vi "Get Ctrl Ref to Connect Unflatten Node.vi"(0 "VI Ref In":refnum<vi>, 5 "JSON String":string, 11 "Error In":errorcluster) -> (4 "Control Terminal References":T1[](array[typedef]), 15 "Error Out":errorcluster)   [LabVIEW 2019, in "JsonToCluster.lvlib"]
doc: "This VI gets control references to connect with unflatten from json string node"
uses:
  JsonToCluster.lvlib
  _Controls/Control Terminal Reference.ctl
  <vilib>/Utility/miscctls.llb/LVPositionTypeDef.ctl
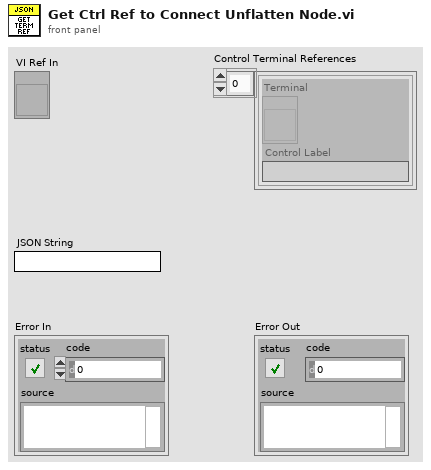
[diagram p1: front panel]
types:
  T1 = typedef "JsonToCluster.lvlib/Control Terminal Reference.ctl" = cluster{"Terminal":refnum<vi>, "Control Label":string}
  T2 = typedef "LVPositionTypeDef.ctl" = cluster{"Left":i32, "Top":i32}
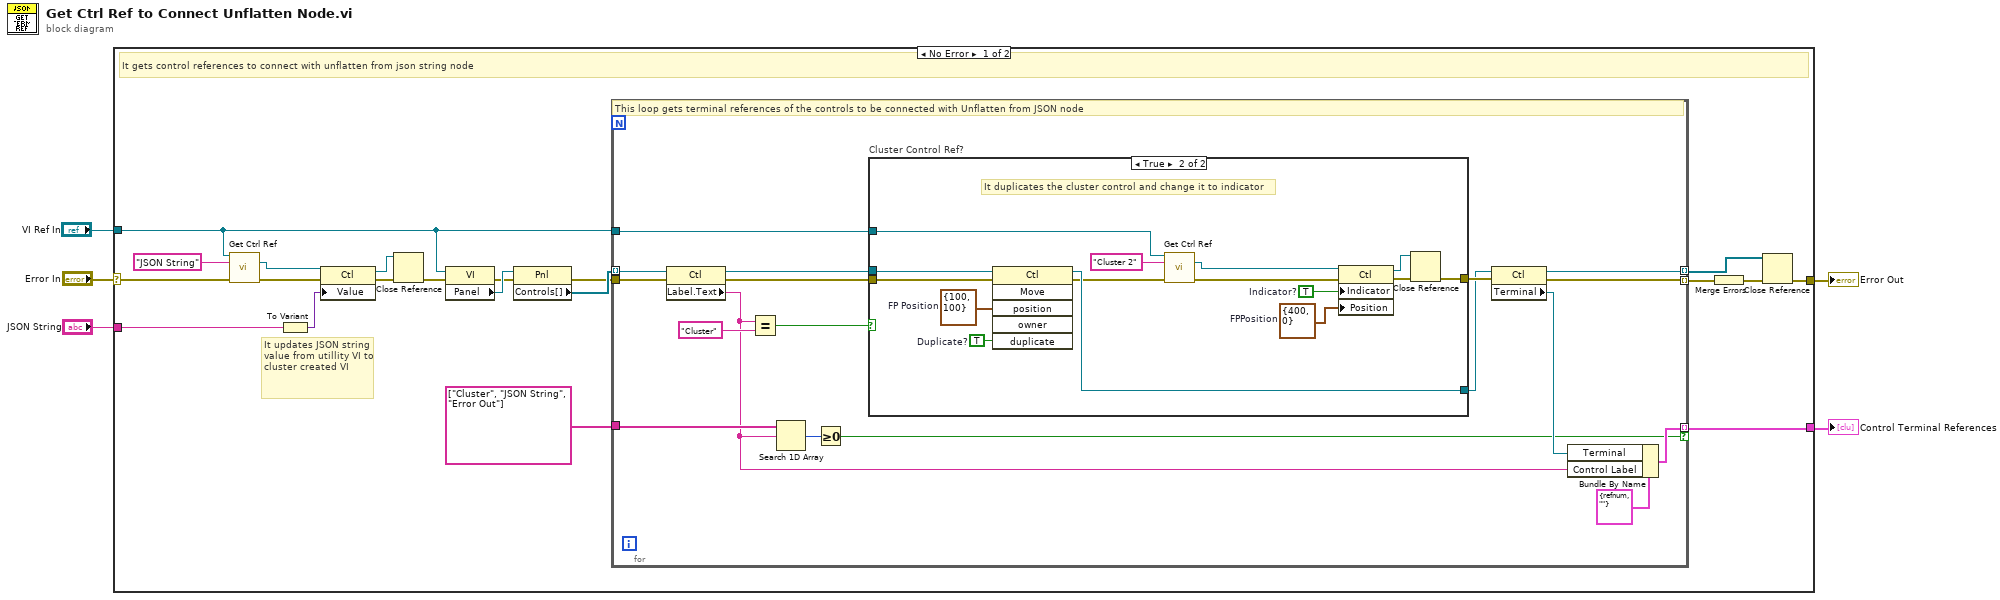
[diagram p0: block diagram]
diagram:
  n1 = case shown="No Error" "Error In" {
    selector: "Error In" -> [w10 w61]
    tunnel: "VI Ref In" -> [w8 _]
    tunnel: "JSON String" -> [w16 _]
    tunnel: [w19 w61] -> w2
    tunnel: [w17 _] -> w1
    frame No Error {
      # "It updates JSON string value from utillity VI to cluster created VI"
      # "It gets control references to connect with unflatten from json string node"
      n2 = call "Get Ctrl Ref.vi"("VI Reference In"=w8, "Control Path"="JSON String", "Error In"=w10) -> ("Ctl Refnum"=w6:refnum<vi>, "Error Out"=w9:errorcluster)  [unwired: 10 in, 1 out]
      n3 = To Variant(anything=w16) -> (Variant=w15:variant)
      n4 = property class="Ctl"(reference=w6, error in=w9, "Value"=w15) -> (reference out=w12:refnum<vi>, error out=w14:errorcluster)
      n5 = Close Reference(reference=w12, error in (no error)=w14) -> (error out=w13:errorcluster)
      n6 = property class="VI"(reference=w8, error in=w13) -> (error out=w20:errorcluster, "Panel"=w21:refnum<vi>)  [unwired: 1 out]
      n7 = property class="Pnl"(reference=w21, error in=w20) -> (error out=w22:errorcluster, "Controls[]"=w23:refnum<vi>[])  [unwired: 1 out]
      n8 = for {
        tunnel: w22 -> [w34]
        tunnel: [w41] -> w24 mode=indexing
        tunnel: w23 -> [w43] mode=indexing
        tunnel: [w30] -> w17 mode=indexing if=w27
        tunnel: w8 -> [w37]
        tunnel: [w33] -> w18 mode=indexing
        tunnel: string[] ["Cluster", "JSON String", "Error Out"] ("y") -> [w29]
        # "This loop gets terminal references of the controls to be connected with Unflatten from JSON node"
        n9 = property class="Ctl"(reference=w43, error in=w34) -> (reference out=w36:refnum<vi>, error out=w40:errorcluster, "Label.Text"=w26:string)
        n10 = Equal?(x=w26, y="Cluster") -> (x = y?=w35:bool)
        n11 = Search 1D Array(1D array=w29, element=w26) -> (index of element=w28:i32)  [unwired: 1 in]
        n12 = Greater Or Equal To 0?(x=w28) -> (x >= 0?=w27:bool)
        n13 = case "Cluster Control Ref?" shown="True" w35 {
          tunnel: w40 -> [w45 w60]
          tunnel: w36 -> [w44 w58]
          tunnel: [w45 w52] -> w39
          tunnel: [w44 w56] -> w38
          tunnel: w37 -> [_ w48]
          frame False {
          }
          frame True {
            w54 = T2 {"Left"=400, "Top"=0}  # FPPosition
            w55 = TRUE  # Indicator?
            w57 = TRUE  # Duplicate?
            w59 = T2 {"Left"=100, "Top"=100}  # FP Position
            # "It duplicates the cluster control and change it to indicator"
            # "It duplicates the cluster control and change it to indicator"
            n14 = invoke class="Ctl" method="Move"(reference=w58, error in=w60, "position"=w59, "duplicate"=w57) -> (reference out=w56:refnum<vi>, error out=w50:errorcluster)  [unwired: 2 in, 4 out]
            n15 = call "Get Ctrl Ref.vi"("VI Reference In"=w48, "Control Path"="Cluster 2", "Error In"=w50) -> ("Ctl Refnum"=w46:refnum<vi>, "Error Out"=w49:errorcluster)  [unwired: 10 in, 1 out]
            n16 = property class="Ctl"(reference=w46, error in=w49, "Indicator"=w55, "Position"=w54) -> (reference out=w51:refnum<vi>, error out=w53:errorcluster)
            n17 = Close Reference(reference=w51, error in (no error)=w53) -> (error out=w52:errorcluster)
          }
        }
        n18 = property class="Ctl"(reference=w38, error in=w39) -> (reference out=w33:refnum<vi>, error out=w41:errorcluster, "Terminal"=w31:refnum<vi>)
        n19 = Bundle By Name(cluster=T1 {"Terminal"=refnum, "Control Label"=""}, "Terminal"=w31, "Control Label"=w26) -> (w30:T1)
      }
      n20 = Merge Errors(w24) -> (w25:errorcluster)
      n21 = Close Reference(reference=w18, error in (no error)=w25) -> (error out=w19:errorcluster)
    }
    frame Error {
      # "If error, this case pass that error message only"
    }
  }
  "Error Out" <- w2
  "Control Terminal References" <- w1
